vi "post_dust_event_big.vi"(8 "error in (no error)":errorcluster, 10 "Signal Array":T1[](array[typedef]), 11 "Cluster":T4 {"File Location" items=["Unknown"=-1, "Processing"=0, "Storage"=1]}) -> (0 "error out":errorcluster, 1 "Experiment Settings":i32, 2 "Dust Event ID":i64, 3 "Test Server":bool)   [LabVIEW 2013]
uses:
  Public API/Post_Dust_Event.ctl
  Controls/File_location.ctl
  Public API/Signal.ctl
  Controls/Role ID.ctl
  Controls/Hardware ID.ctl
  NaN_screening_big.vi
  <vilib>/addons/database/_DB Variant To Data/Database Variant To Data.xnode
  <vilib>/addons/database/NI_Database_API.lvlib
panel:
  # "Signal"
  # "Dust Event"
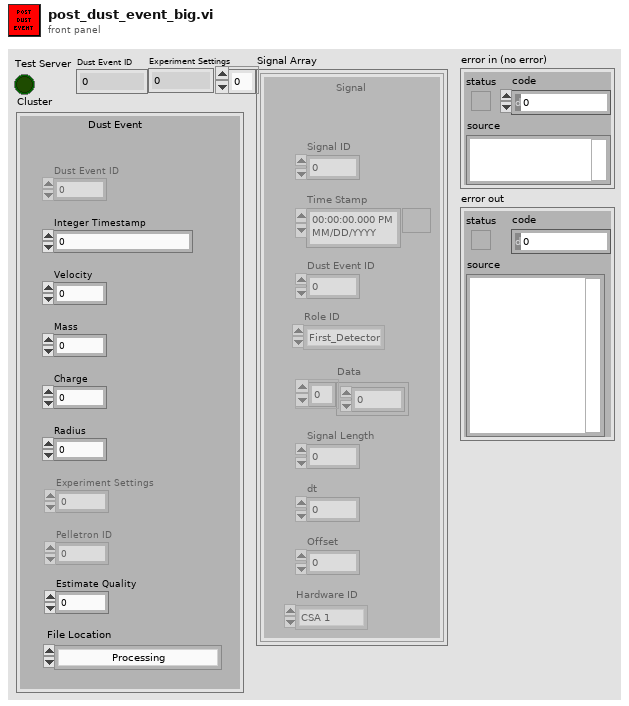
[diagram p1: front panel]
types:
  T1 = typedef "Signal.ctl" = cluster{"Signal ID":i64, "Time Stamp":timestamp, "Dust Event ID":i64, "Role ID":T2, "Data":sgl[], "Signal Length":i32, "dt":sgl, "Offset":dbl, "Hardware ID":T3}
  T2 = typedef "Role ID.ctl" = enum16{"First_Detector", "Second_Detector", "Third_Detector", "LeCroy_CH1", "LeCroy_CH2", "LeCroy_CH3", "LeCroy_CH4", "PSU"}
  T3 = typedef "Hardware ID.ctl" = enum16{"Unknown", "CSA 1", "CSA 2", "CSA 3", "CSA 4", "CSA 5", "CSA 6"}
  T4 = typedef "Post_Dust_Event.ctl" = cluster{"Dust Event ID":i64, "Integer Timestamp":i64, "Velocity":sgl, "Mass":sgl, "Charge":sgl, "Radius":sgl, "Experiment Settings":dbl, "Pelletron ID":i32, "Estimate Quality":sgl, "File Location":T5, "id_dust_info":dbl}
  T5 = typedef "File_location.ctl" = i8
  T6 = typedef "NI_Database_API.lvlib/Conn ObjectReference.ctl" = refnum<k1>
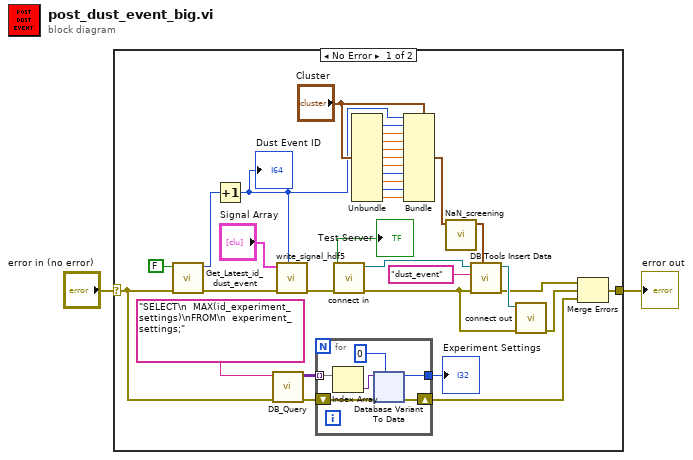
[diagram p0: block diagram]
diagram:
  n1 = case shown="No Error" "error in (no error)" {
    selector: "error in (no error)" -> [w4 w74]
    tunnel: [w35 w74] -> w1
    frame No Error {
      n2 = call "Get_Latest_id_dust_event.vi"("error in (no error)"=w4, "Small?"=FALSE) -> ("error out"=w14:errorcluster, "id_dust_event"=w13:i64)  [unwired: 8 in]
      n3 = Increment(x=w13) -> (x+1=w18:i64)
      "Dust Event ID" <- w18
      n4 = call "DB_Query.vi"("error in (no error)"=w4, "Parameterized Query"="SELECT\n  MAX(id_experiment_settings)\nFROM\n  experiment_settings;" ("SQL query")) -> ("error out"=w7:errorcluster, "Results"=w5:variant[][])  [unwired: 7 in, 1 out]
      n5 = call "write_signal_hdf5.vi"("Index"=w18, "error in"=w14, "Signal array"="Signal Array") -> ("error out"=w12:errorcluster)  [unwired: 7 in, 1 out]
      n6 = for {
        tunnel: [w39] -> w16
        shift-right: [w37] -> w6
        shift-left: w7 -> [w38]
        tunnel: w5 -> [w36] mode=indexing
        n7 = Index Array(array=w36) -> (element=w41:variant)  [unwired: 1 in]
        n8 = xnode "Database Variant To Data"("database variant"=w41, "error in (no error)"=w38, "type"=0) -> ("data"=w39:i32, "error out"=w37:errorcluster)
      }
      "Experiment Settings" <- w16
      n9 = call "connect in.vi"("error in (no error)"=w12) -> ("error out"=w9:errorcluster, "Database Connection"=w11:T6, "Test Server"=→"Test Server":bool)  [unwired: 6 in]
      n10 = Unbundle("Cluster") -> ("Integer Timestamp"=w19:i64, "Velocity"=w20:sgl, "Mass"=w21:sgl, "Charge"=w22:sgl, "Radius"=w23:sgl, "Experiment Settings"=w24:dbl, "Pelletron ID"=w25:i32, "Estimate Quality"=w26:sgl, "File Location"=w17:T5, "id_dust_info"=w27:dbl)  [unwired: 1 out]
      n11 = Bundle(cluster="Cluster", "Dust Event ID"=w18, "Integer Timestamp"=w19, "Velocity"=w20, "Mass"=w21, "Charge"=w22, "Radius"=w23, "Experiment Settings"=w24, "Pelletron ID"=w25, "Estimate Quality"=w26, "File Location"=w17, "id_dust_info"=w27) -> (w28:T4)
      n12 = call-poly "NaN_screening.vi"("Input"=w28) -> ("Output"=w34:T4)  [unwired: 10 in]
      n13 = call <vilib>:"DB Tools Insert Data.vi"("data"=w34, "error in (no error)"=w9, "table"="dust_event", "connection reference"=w11) -> ("error out"=w30:errorcluster, "connection reference out"=w31:T6)  [unwired: 6 in]
      n14 = call "connect out.vi"("error in (no error)"=w9, "connection reference"=w31) -> ("error out"=w15:errorcluster)  [unwired: 9 in]
      n15 = Merge Errors(w30, w15, w6) -> (w35:errorcluster)
    }
    frame Error {
    }
  }
  "error out" <- w1
